vi "UE9 Multiple EI-1050 Example.vi"() -> ()   [LabVIEW 2021]
panel:
  in  "B Enable Channel":i32=4
  in  "A Enable Channel":i32=3
  in  "Power Channel":i32=2
  in  "Clock Channel":i32=1
  in  "Data Channel":i32
  in  "stop":bool
  out "ms per iteration":u32
  out "RH B [%]":dbl format="%.6f"
  out "RH A [%]":dbl format="%.6f"
  out "Temp B [degC]":dbl format="%.6f"
  out "Temp A [degC]":dbl format="%.6f"
  out "Error Message":string
  out "error out":errorcluster
  # "Reads temperature and humidity\nfrom a pair of EI-1050 probes:\n\nBoth Probes:\nRed (Power)         FIO2\nBlack (Ground)     GND\nGreen (Data)        FIO0\nWhite (Clock)       FIO1\n\n\n\n\n\nProbe A:\nBrown (Enable)    FIO3\n\nProbe B:\nBrown (Enable)    FIO4"
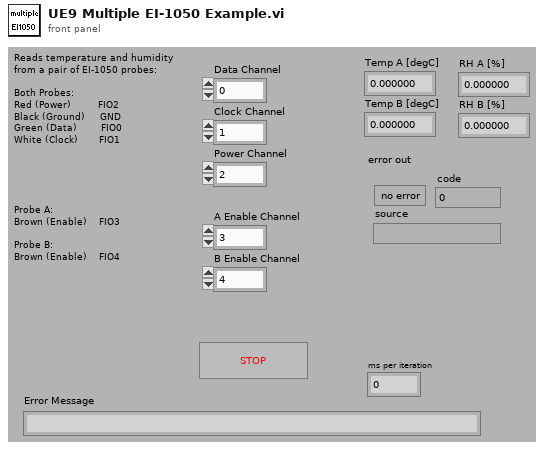
[diagram p1: front panel]
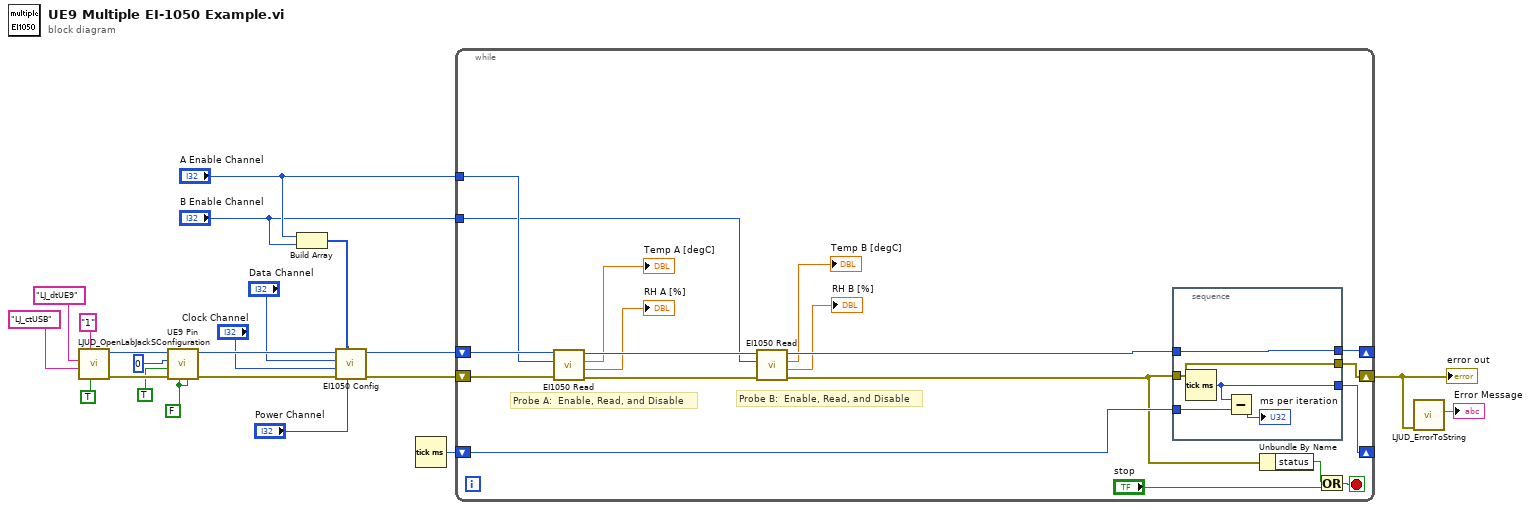
[diagram p0: block diagram]
diagram:
  w12 = FALSE ("Enable DAC1")
  n1 = call "LJUD_OpenLabJackS.vi"("FirstFound"=TRUE, "Address"="1", "ConnectionType"="LJ_ctUSB", "DeviceType"="LJ_dtUE9") -> ("error out"=w16:errorcluster, "Handle"=w17:i32)  [unwired: 5 in, 1 out]
  n2 = call "UE9 Pin Configuration.vi"("Enable Counter1"=w12, "Enable Counter0"=w12, "error in"=w16, "Enable DACs"=TRUE ("Enable DAC1"), "Number of Timers Enabled"=u8 0, "Handle In"=w17) -> ("error out"=w9:errorcluster, "Handle Out"=w10:i32)  [unwired: 4 in]
  n3 = Build Array("A Enable Channel", "B Enable Channel") -> (w3:i32[])
  n4 = call "EI1050 Config.vi"("Power Channel"="Power Channel", "Enable Channels"=w3, "error in"=w9, "Clock Channel"="Clock Channel", "Data Channel"="Data Channel", "Handle In"=w10) -> ("error out"=w7:errorcluster, "Handle Out"=w8:i32)  [unwired: 4 in]
  n5 = Tick Count (ms)() -> (millisecond timer value=w14:u32)
  n6 = while {
    tunnel: "B Enable Channel" -> [w23]
    tunnel: "A Enable Channel" -> [w24]
    shift-left: w14 -> [w38]
    shift-right: [w41] -> _
    shift-left: w8 -> [w34]
    shift-right: [w39] -> _
    shift-left: w7 -> [w33]
    shift-right: [w40] -> w13
    stop <- w37 stop-if-true
    # "Probe A:  Enable, Read, and Disable"
    # "Probe B:  Enable, Read, and Disable"
    n7 = call "EI1050 Read.vi"("error in"=w33, "Enable Channel (or -1)"=w24, "Handle In"=w34) -> ("error out"=w31:errorcluster, "RH [%]"=→"RH A [%]":dbl, "Temp [degC]"=→"Temp A [degC]":dbl, "Handle Out"=w32:i32)  [unwired: 4 in, 1 out]
    n8 = call "EI1050 Read.vi"("error in"=w31, "Enable Channel (or -1)"=w23, "Handle In"=w32) -> ("error out"=w29:errorcluster, "RH [%]"=→"RH B [%]":dbl, "Temp [degC]"=→"Temp B [degC]":dbl, "Handle Out"=w30:i32)  [unwired: 4 in, 1 out]
    n9 = stacked-sequence {
      tunnel: [w46] -> w41
      tunnel: w29 -> [w45]
      tunnel: [w45] -> w40
      tunnel: [w44] -> w39
      tunnel: w30 -> [w44]
      tunnel: w38 -> [w43]
      frame #0 {
        n10 = Tick Count (ms)() -> (millisecond timer value=w46:u32)
        n11 = Subtract(x=w46, y=w43) -> (x-y=→"ms per iteration":u32)
      }
    }
    n12 = Unbundle By Name(w29) -> ("status"=w36:bool)
    n13 = Or(x=w36, y="stop") -> (x .or. y?=w37:bool)
  }
  "error out" <- w13
  n14 = call "LJUD_ErrorToString.vi"("error in"=w13) -> ("String"=→"Error Message":string)  [unwired: 10 in]
